vi "Iniciar Adquisicion.vi"(8 "error in (no error)":errorcluster, 11 "Camara in":refnum<class "Camara.lvclass">) -> (0 "error out":errorcluster, 3 "Camara out":refnum<class "Camara.lvclass">)   [LabVIEW 2020, in "Camara.lvclass"]
uses:
  Camara.lvclass
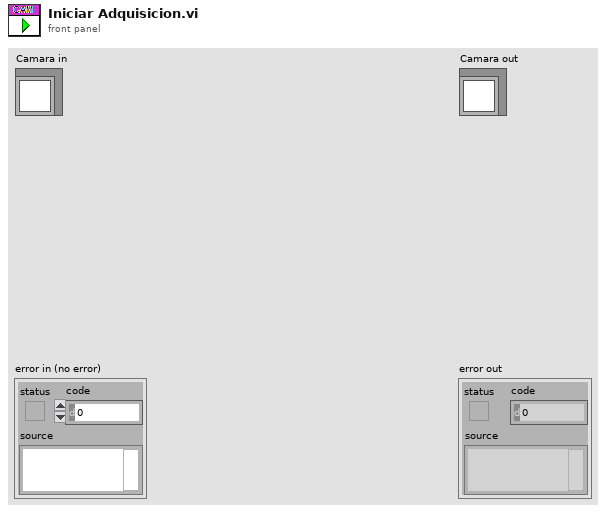
[diagram p1: front panel]
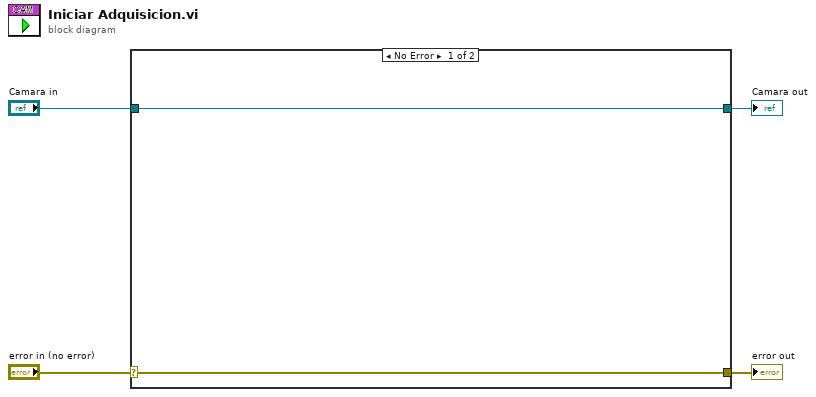
[diagram p0: block diagram]
diagram:
  n1 = case shown="No Error" "error in (no error)" {
    selector: "error in (no error)" -> [w5 w8]
    tunnel: [w5 w8] -> w3
    tunnel: [w6 w7] -> w1
    tunnel: "Camara in" -> [w6 w7]
    frame No Error {
    }
    frame Error {
    }
  }
  "error out" <- w3
  "Camara out" <- w1
